vi "Set Zero Offset.vi"(8 "error in (no error)":errorcluster, 9 "(in/out)put":enum16{"Input", "Output"}(ring), 10 "Offset":dbl min=-20.0 max=80.0, 11 "EXFO in":refnum<class "EXFO.lvclass">) -> (0 "error out":errorcluster, 3 "EXFO out":refnum<class "EXFO.lvclass">)   [LabVIEW 2018, in "LTB-1.lvlib" / "LTB-1.lvclass"]
uses:
  LTB-1.lvclass
  PPLs/EXFO/Parent/EXFO.lvlibp/EXFO.lvclass
  PPLs/EXFO/Parent/EXFO.lvlibp/Methods/Read Resource.vi
  3150 Driver/3150.lvlib
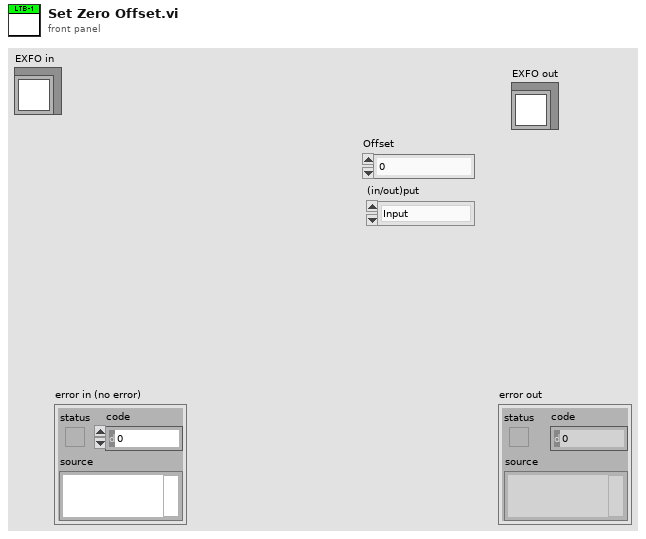
[diagram p1: front panel]
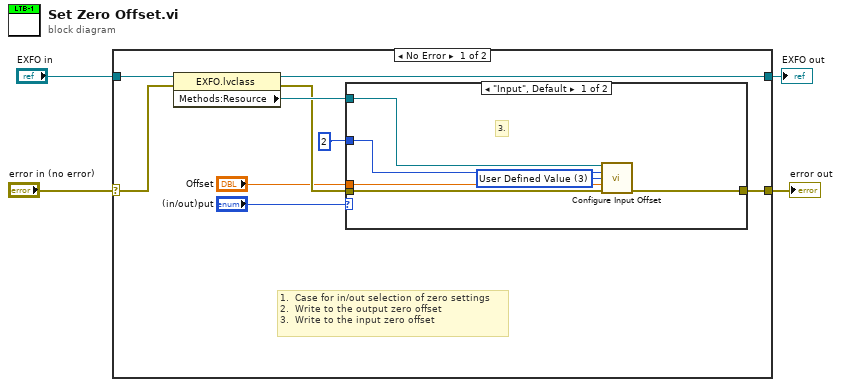
[diagram p0: block diagram]
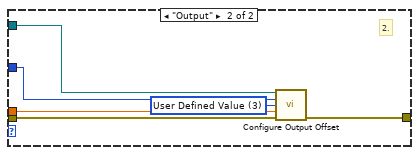
[diagram p2: hidden frame]
diagram:
  n1 = case shown="No Error" "error in (no error)" {
    selector: "error in (no error)" -> [w11 w27]
    tunnel: [w10 w27] -> w3
    tunnel: [w12 w26] -> w1
    tunnel: "EXFO in" -> [w13 w26]
    frame No Error {
      # "1.  Case for in/out selection of zero settings\n2.  Write to the output zero offset\n3.  Write to the input zero offset"
      n2 = property class="EXFO.lvclass"(reference=w13, error in=w11) -> (reference out=w12:refnum<class "EXFO.lvclass">, error out=w6:errorcluster, "Methods:Resource"=w8:refnum<visa-resource-name>)
      n3 = case shown="\"Input\", Default" "(in/out)put" {
        tunnel: w6 -> [w16 w22]
        tunnel: [w15 w21] -> w10
        tunnel: w8 -> [w19 w25]
        tunnel: i16 2 ("Module Slot Number (10)") -> [w18 w24]
        tunnel: "Offset" -> [w17 w23]
        frame "Input", Default {
          w14 = u16 3 items=["MINimum", "MAXimum", "DEFault", "User Defined Value"] ("Input Offset (0:MINimum)")
          # "3."
          n4 = call "Configure Input Offset.vi"("VISA resource name"=w19, "Platform Slot Number (10)"=w18, "Input Offset (0:MINimum)"=w14, "User Defined Offset Value (-5.000)"=w17, "error in (no error)"=w16) -> ("error out"=w15:errorcluster)  [unwired: 9 in, 1 out]
        }
        frame "Output" {
          w20 = 3 items=["MINimum", "MAXimum", "DEFault", "User Defined Value"] ("Output Offset (0:MINimum)")
          # "2."
          n5 = call "Configure Output Offset.vi"("VISA resource name"=w25, "Platform Slot Number (10)"=w24, "Output Offset (0:MINimum)"=w20, "User Defined Output Offset Value (-1.500)"=w23, "error in (no error)"=w22) -> ("error out"=w21:errorcluster)  [unwired: 9 in, 1 out]
        }
      }
    }
    frame Error {
    }
  }
  "error out" <- w3
  "EXFO out" <- w1
